vi "闹钟（多次时分秒）.vi"(5 "设置时间":i32[](array[numeric]) format="%< %H-%M-%S>t", 7 "启用":bool=TRUE) -> (6 "时间到脉冲":bool, 8 "当前时分秒":i32 format="%< %H-%M-%S>t")   [LabVIEW 2012]
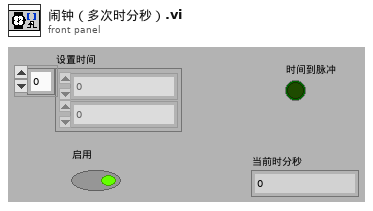
[diagram p1: front panel]
types:
  T1 = typedef "LVDateTimeRec.ctl" = cluster{"秒数的小数部分":dbl, "秒":i32, "分":i32, "时":i32, "日":i32, "月":i32, "年":i32, "天数（周）":i32, "天数（年）":i32, "DST":i32}
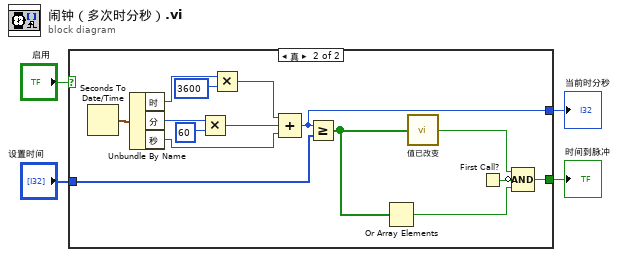
[diagram p0: block diagram]
diagram:
  n1 = case shown="真" "启用" {
    tunnel: "设置时间" -> [_ w17]
    tunnel: [_ w19] -> w2
    tunnel: [_ w5] -> w1
    frame False {
    }
    frame True {
      n2 = Seconds To Date/Time() -> (date time rec=w6:T1)  [unwired: 2 in]
      n3 = Unbundle By Name(w6) -> ("时"=w7:i32, "分"=w9:i32, "秒"=w13:i32)
      n4 = Multiply(x=w9, y=60) -> (x*y=w11:i32)
      n5 = Multiply(x=w7, y=3600) -> (x*y=w12:i32)
      n6 = Compound Arithmetic op=ADD(w12, w11, w13) -> (w5:i32)
      n7 = Greater Or Equal?(x=w5, y=w17) -> (x >= y?=w15:bool[])
      n8 = Or Array Elements(Boolean array=w15) -> (logical OR=w14:bool)
      n9 = call-poly "值已改变.vi"("输入数据"=w15) -> ("已更改"=w16:bool)  [unwired: 3 in]
      n10 = First Call?() -> (First Call?: T/F=w18:bool)
      n11 = Compound Arithmetic op=AND(w16, invert w18, w14) -> (w19:bool)
    }
  }
  "时间到脉冲" <- w2
  "当前时分秒" <- w1
